vi "Link Message Parameters.vi"(8 "error in (no error)":errorcluster, 10 "Starting Address":u16 format="%04x", 11 "Message in":refnum<class "Message.lvclass">) -> (0 "error out":errorcluster, 3 "Message out":refnum<class "Message.lvclass">)   [LabVIEW 2020, in "BCI-1553 API.lvlib" / "Message.lvclass"]
doc: "Links each parameter for this message to an address. This will be recalled by the bus controller at a later time to setup quick parameter retrieval mechanisms."
uses:
  Message.lvclass
  Message.lvclass/Message.ctl
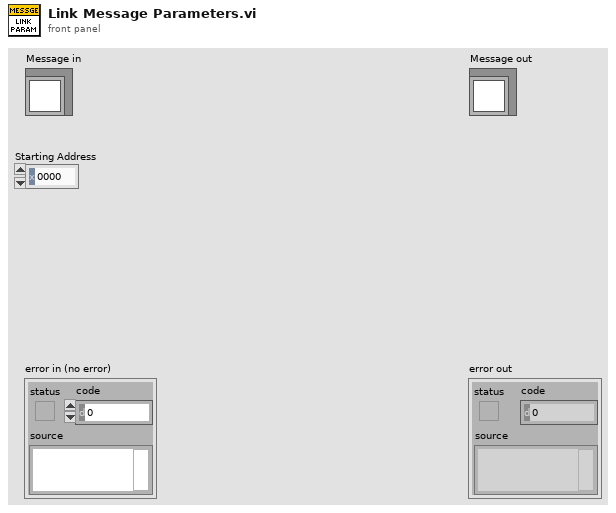
[diagram p1: front panel]
types:
  T1 = typedef "BCI-1553 API.lvlib/Parameter Table Data.ctl" = cluster{"Parameter Name":string, "Base Word":u16, "Address":u16, "Value":u64, "Mask":u16[], "Scaling Info":T2}
  T2 = typedef "BCI-1553 API.lvlib/Scaling Information.ctl" = cluster{"Bit Offset":i32, "Bit Count":i32, "LSB Resolution":dbl, "2's Complement":bool, "Big Endian":bool, "Sign Bit":bool}
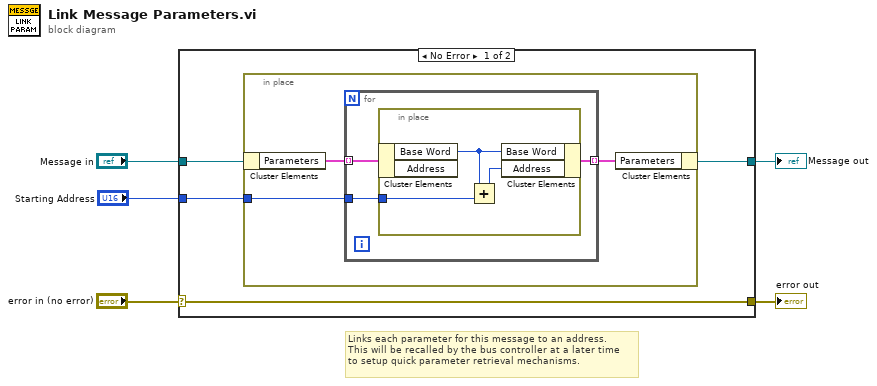
[diagram p0: block diagram]
diagram:
  # "Links each parameter for this message to an address.\nThis will be recalled by the bus controller at a later time\nto setup quick parameter retrieval mechanisms."
  n1 = case shown="No Error" "error in (no error)" {
    selector: "error in (no error)" -> [w9 w20]
    tunnel: [w9 w20] -> w4
    tunnel: [w7 w19] -> w2
    tunnel: "Message in" -> [w8 w19]
    tunnel: "Starting Address" -> [w6 _]
    frame No Error {
      n2 = in-place {
        in-place-border: w6 -> [w11]
        n3 = in-place-cluster #1(w8) -> ("Parameters"=w12:T1[])
        n4 = for {
          tunnel: w12 -> [w15] mode=indexing
          tunnel: w11 -> [w14]
          tunnel: [w13] -> w10 mode=indexing
          n5 = in-place {
            in-place-border: w14 -> [w18]
            n6 = in-place-cluster #2(w15) -> ("Base Word"=w16:u16)  [unwired: 1 out]
            n7 = Add(x=w16, y=w18) -> (x+y=w17:u16)
            n8 = in-place-cluster #2("Base Word"=w16, "Address"=w17) -> (w13:T1)
          }
        }
        n9 = in-place-cluster #1("Parameters"=w10) -> (w7:refnum<class "Message.lvclass">)
      }
    }
    frame Error {
    }
  }
  "error out" <- w4
  "Message out" <- w2
